vi "TCP Read.vi"(7 "mode (standard)":T1(ring), 8 "error in (no error)":errorcluster, 10 "bytes to read":i32, 11 "TCP in":refnum<class "TCP.lvclass">) -> (0 "error out":errorcluster, 1 "timed out?":bool, 2 "data":string, 3 "TCP out":refnum<class "TCP.lvclass">)   [LabVIEW 2021, in "TCP.lvclass"]
doc: "Reads from the established TCP connection stored in the class."
uses:
  TCP.lvclass
  TCP.lvclass/TCP.ctl
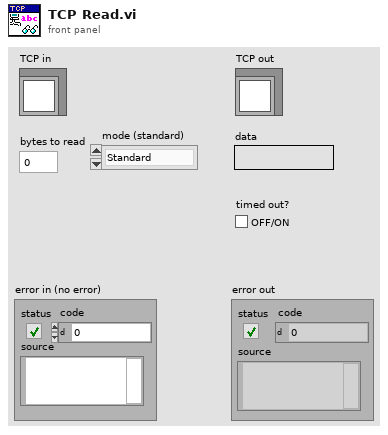
[diagram p1: front panel]
types:
  T1 = enum16{"Standard", "Buffered", "CRLF", "Immediate"}
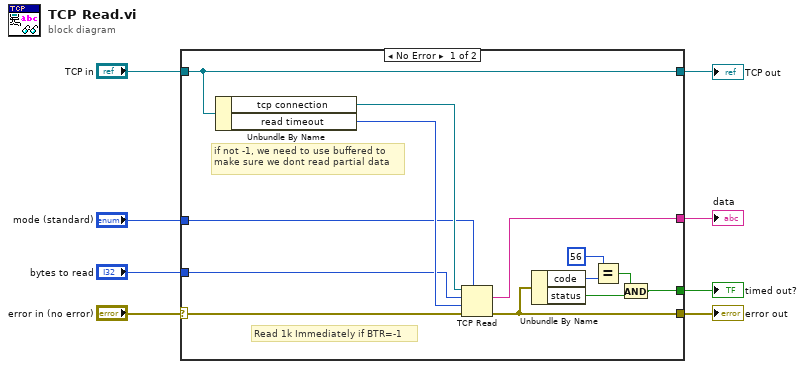
[diagram p0: block diagram]
diagram:
  n1 = case shown="No Error" "error in (no error)" {
    selector: "error in (no error)" -> [w20 w23]
    tunnel: [w21 w23] -> w6
    tunnel: "bytes to read" -> [w11 _]
    tunnel: [w9 _] -> w5
    tunnel: "TCP in" -> [w15 w22]
    tunnel: [w15 w22] -> w3
    tunnel: [w12 _] -> w2
    tunnel: "mode (standard)" -> [w10 _]
    frame No Error {
      # "Read 1k Immediately if BTR=-1"
      # "if not -1, we need to use buffered to\nmake sure we dont read partial data"
      n2 = Unbundle By Name(w15) -> ("tcp connection"=w14:refnum<k5>, "read timeout"=w13:i32)
      n3 = TCP Read(connection ID=w14, bytes to read=w11, error in (no error)=w20, 7:w10, 9:w13) -> (data out=w12:string, error out=w21:errorcluster)  [unwired: 1 out]
      n4 = Unbundle By Name(w21) -> ("code"=w19:i32, "status"=w16:bool)
      n5 = Equal?(x=56, y=w19) -> (x = y?=w17:bool)
      n6 = And(x=w17, y=w16) -> (x .and. y?=w9:bool)
    }
    frame Error {
    }
  }
  "error out" <- w6
  "TCP out" <- w3
  "timed out?" <- w5
  "data" <- w2
